vi "test weight projected images.vi"() -> ()   [LabVIEW 2010]
panel:
  out "m2 out":u16[][](array[numeric])
  out "m1 out":u16[][](array[numeric])
  in  "m2":u16[][](array[numeric])=[[3, 3, 3], [3, 3, 3], [3, 3, 3]]
  in  "m1":u16[][](array[numeric])=[[1, 2, 3], [4, 5, 6], [7, 8, 9]]
  in  "num frames":u8=2
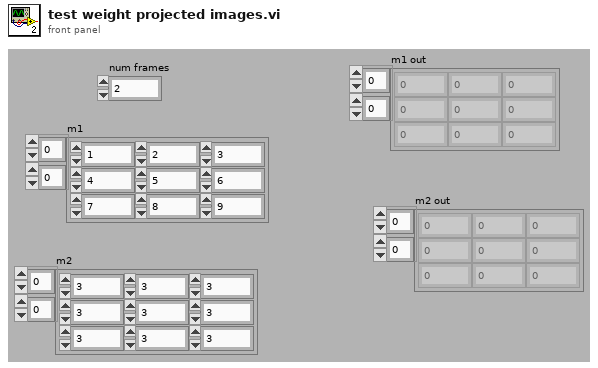
[diagram p1: front panel]
types:
  T1 = cluster{"xy ch 0":u16[][], "xy ch 1":u16[][], "zx ch0":u16[][], "zx ch1":u16[][], "zy ch0":u16[][], "zy ch1":u16[][], "zx ch0 fb":u16[][], "zx ch1fb":u16[][], "zy ch0 fb":u16[][], "zy ch1 fb":u16[][]}
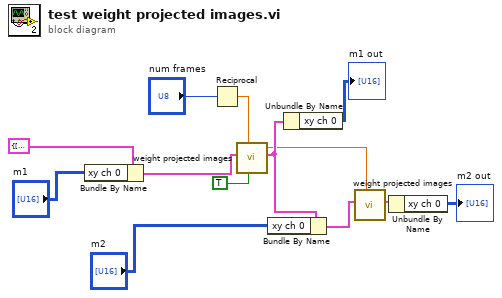
[diagram p0: block diagram]
diagram:
  n1 = Bundle By Name(cluster=T1 {"xy ch 0"=[], "xy ch 1"=[], "zx ch0"=[], "zx ch1"=[], "zy ch0"=[], "zy ch1"=[], "zx ch0 fb"=[], "zx ch1fb"=[], "zy ch0 fb"=[], "zy ch1 fb"=[]} ("projections"), "xy ch 0"="m1") -> (w8:T1)
  n2 = Reciprocal(x="num frames") -> (1/x=w1:dbl)
  n3 = call "weight projected images.vi"("reset?"=TRUE, "weight"=w1, "projections"=w8) -> ("projections out"=w2:T1)  [unwired: 6 in, 2 out]
  n4 = Bundle By Name(cluster=w2, "xy ch 0"="m2") -> (w6:T1)
  n5 = Unbundle By Name(w2) -> ("xy ch 0"=→"m1 out":u16[][])
  n6 = call "weight projected images.vi"("weight"=w1, "projections"=w6) -> ("projections out"=w4:T1)  [unwired: 7 in, 2 out]
  n7 = Unbundle By Name(w4) -> ("xy ch 0"=→"m2 out":u16[][])
